vi "Main.vi"() -> ()   [LabVIEW 2024]
panel:
  out "OUTPUTS":T1
  out "INPUTS":T2
  out "Output Lockout Status":bool
  out "Output over current alert Ch I2T Levels":T3
  out "Cluster 2":T4
  out "Switching Card \nFirmware Version":T5
  out "Control Card \nConfiguration Version":T6 {"Major Version" format="%.0x"; "Minor Version" format="%.0x"}
  out "Control Card \nFirmware Version":T5
  out "Cluster":T7
  in  "Channel Number":dbl
  in  "Card Number":dbl
  in  "String":string
  in  "send":bool
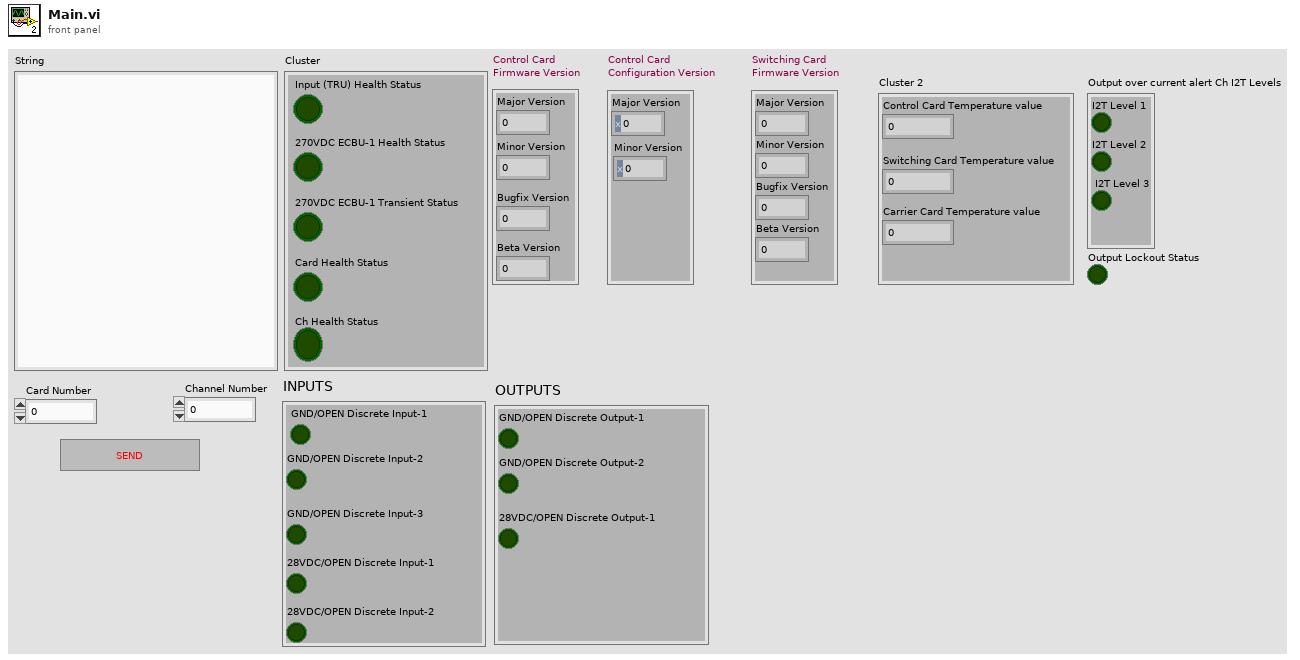
[diagram p1: front panel]
types:
  T1 = cluster{"GND/OPEN Discrete Output-1 ":bool, "GND/OPEN Discrete Output-2":bool, "28VDC/OPEN Discrete Output-1":bool}
  T2 = cluster{"GND/OPEN Discrete Input-1":bool, "GND/OPEN Discrete Input-2":bool, "GND/OPEN Discrete Input-3":bool, "28VDC/OPEN Discrete Input-1":bool, "28VDC/OPEN Discrete Input-2":bool}
  T3 = cluster{"I2T Level 1":bool, "I2T Level 2":bool, " I2T Level 3":bool}
  T4 = cluster{"Control Card Temperature value ":dbl, "Switching Card Temperature value":dbl, "Carrier Card Temperature value":dbl}
  T5 = cluster{"Major Version":u16, "Minor Version":u16, "Bugfix Version":u16, "Beta Version":u16}
  T6 = cluster{"Minor Version":u16, "Major Version":u16}
  T7 = cluster{"270VDC ECBU-1 Health Status":bool, "270VDC ECBU-1 Transient Status":bool, "Input (TRU) Health Status":bool, "Card Health Status":bool, "Ch Health Status":bool}
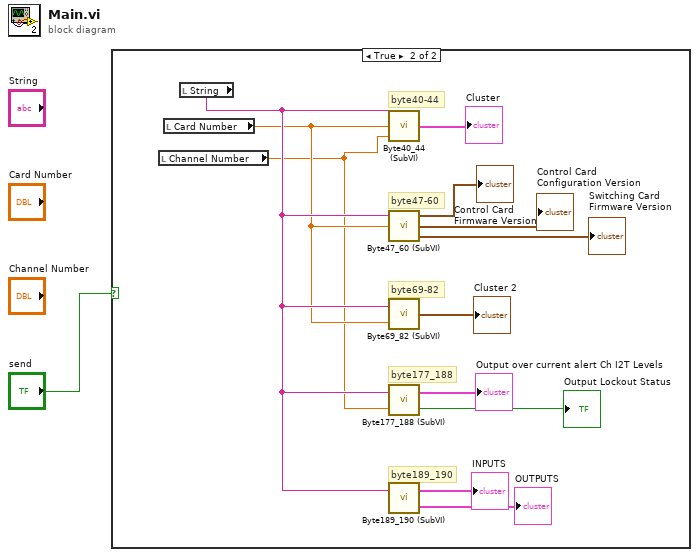
[diagram p0: block diagram]
diagram:
  n1 = case shown="True" "send" {
    frame False {
    }
    frame True {
      # "byte189_190"
      # "byte177_188"
      # "byte69-82"
      # "byte47-60"
      # "byte40-44"
      n2 = local read "Channel Number"() -> (w11:dbl)
      n3 = local read "Card Number"() -> (w12:dbl)
      n4 = local read "String"() -> (w13:string)
      n5 = call "Byte40_44 (SubVI).vi"("Channel Number"=w11, "Card Number"=w12, "Input String 2"=w13) -> ("Cluster"=→"Cluster":T7)  [unwired: 2 in]
      n6 = call "Byte47_60 (SubVI).vi"("Card Number"=w12, "Input String"=w13) -> ("Switching Card \nFirmware Version"=→"Switching Card \nFirmware Version":T5, "Control Card \nConfiguration Version"=→"Control Card \nConfiguration Version":T6, "Control Card \nFirmware Version"=→"Control Card \nFirmware Version":T5)  [unwired: 1 in]
      n7 = call "Byte69_82 (SubVI).vi"("Card Number"=w12, "Input String"=w13) -> ("Cluster"=→"Cluster 2":T4)
      n8 = call "Byte177_188 (SubVI).vi"("Channel Number"=w11, "Input String"=w13) -> ("Output Lockout Status"=→"Output Lockout Status":bool, "Output over current alert Ch I2T Levels"=→"Output over current alert Ch I2T Levels":T3)
      n9 = call "Byte189_190 (SubVI).vi"("Input String"=w13) -> ("OUTPUTS"=→"OUTPUTS":T1, "INPUTS"=→"INPUTS":T2)  [unwired: 1 in]
    }
  }
